vi "sslSimulationProtocolRobotMoveCommand.vi"(8 "error in (no error)":errorcluster, 10 "robot":T1, 11 "Communication in":refnum<class "Communication.lvclass">) -> (0 "error out":errorcluster, 1 "robotMoveCommand":u8[](array[numeric]), 3 "Communication out":refnum<class "Communication.lvclass">)   [LabVIEW 2023, in "Communication.lvclass"]
uses:
  Communication.lvclass
  Convert AI Robot to Robot Command Folder/grSim/grSim Robot Command.ctl
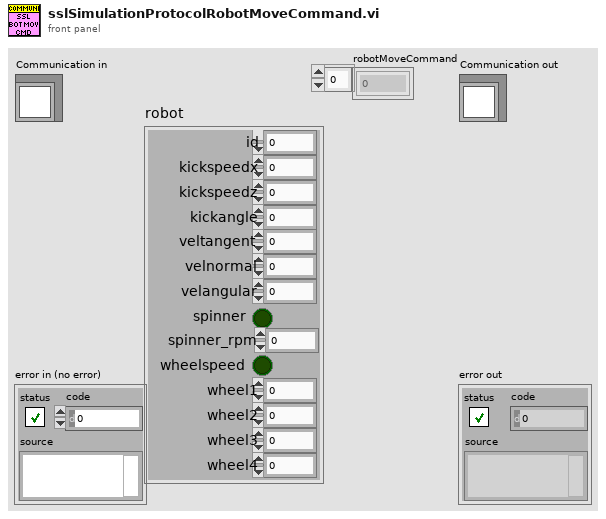
[diagram p1: front panel]
types:
  T1 = typedef "grSim Robot Command.ctl" = cluster{"id":u32, "kickspeedx":sgl, "kickspeedz":sgl, "veltangent":sgl, "velnormal":sgl, "velangular":sgl, "spinner":bool, "wheelspeed":bool, "wheel1":sgl, "wheel2":sgl, "wheel3":sgl, "wheel4":sgl, "kickangle":sgl, "spinner_rpm":sgl}
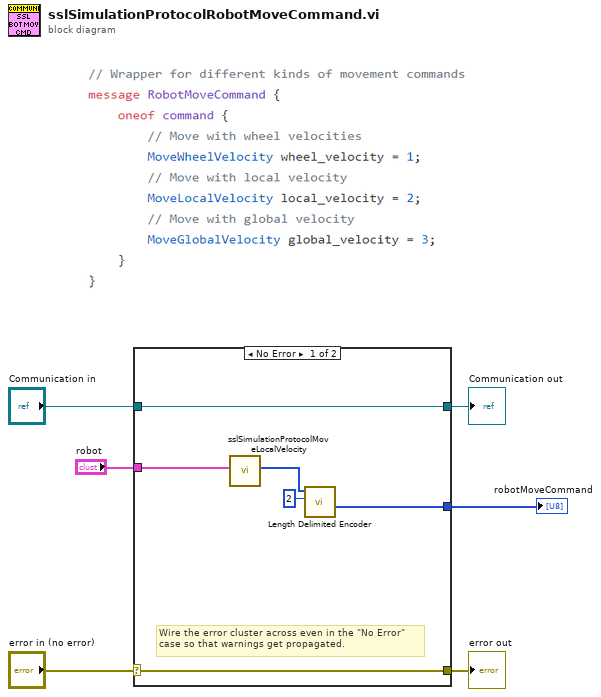
[diagram p0: block diagram]
diagram:
  n1 = case shown="No Error" "error in (no error)" {
    selector: "error in (no error)" -> [w11 w14]
    tunnel: [w11 w14] -> w5
    tunnel: [w12 w13] -> w3
    tunnel: "Communication in" -> [w12 w13]
    tunnel: [w9 _] -> w2
    tunnel: "robot" -> [w7 _]
    frame No Error {
      # "Wire the error cluster across even in the \"No Error\"\ncase so that warnings get propagated."
      n2 = call "sslSimulationProtocolMoveLocalVelocity.vi"("robot"=w7) -> ("MoveLocalVelocity"=w8:u8[])  [unwired: 8 in, 2 out]
      n3 = call "Length Delimited Encoder.vi"("Key"=u32 2, "Array In to be added"=w8) -> ("Array"=w9:u8[])  [unwired: 9 in]
    }
    frame Error {
    }
  }
  "error out" <- w5
  "Communication out" <- w3
  "robotMoveCommand" <- w2
